vi "Sort 2D Array.vi"(8 "error in (no error)":errorcluster, 11 "Array in":string[][](array[string])) -> (0 "error out":errorcluster, 3 "Array out":string[][](array[string]))   [LabVIEW 2025, in "Project.lvclass"]
uses:
  Project.lvclass
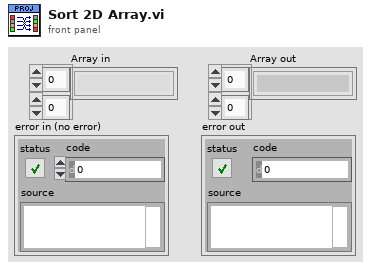
[diagram p1: front panel]
types:
  T1 = typedef "Project.lvclass/FPGA Settings.ctl" = cluster{"FPGA Target Name":string, "Modules":T2[]}
  T2 = typedef "Module.lvclass/Module Settings.ctl" = cluster{"Group Name":string, "Model Number":string, "Signals":T3[]}
  T3 = typedef "Signal.lvclass/Signal Settings.ctl" = cluster{"Signal Name":string, "IO Name":string, "Signal Type":string, "Signal Parameters":string, "IO Resource":string}
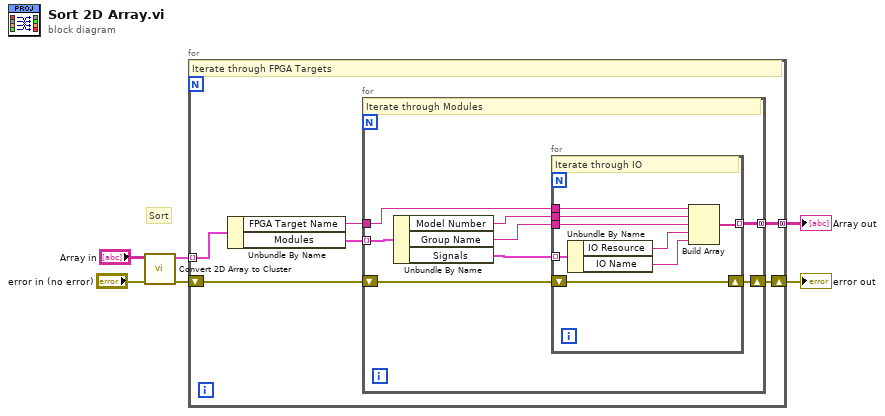
[diagram p0: block diagram]
diagram:
  # "Sort"
  n1 = call "Convert 2D Array to Cluster.vi"("error in (no error)"="error in (no error)", "Array in"="Array in") -> ("error out"=w3:errorcluster, "Array out"=w5:T1[])  [unwired: 8 in]
  n2 = for {
    tunnel: w5 -> [w10] mode=indexing
    shift-right: [w9] -> w1
    shift-left: w3 -> [w11]
    tunnel: [w7] -> w2 mode=concatenating
    # "Iterate through FPGA Targets"
    n3 = Unbundle By Name(w10) -> ("FPGA Target Name"=w8:string, "Modules"=w12:T2[])
    n4 = for {
      tunnel: w12 -> [w19] mode=indexing
      shift-right: [w18] -> w9
      shift-left: w11 -> [w13]
      tunnel: w8 -> [w17]
      tunnel: [w14] -> w7 mode=concatenating
      # "Iterate through Modules"
      n5 = Unbundle By Name(w19) -> ("Model Number"=w16:string, "Group Name"=w15:string, "Signals"=w20:T3[])
      n6 = for {
        tunnel: w20 -> [w21] mode=indexing
        shift-right: [w28] -> w18
        shift-left: w13 -> [w28]
        tunnel: w17 -> [w27]
        tunnel: w16 -> [w26]
        tunnel: w15 -> [w25]
        tunnel: [w22] -> w14 mode=indexing
        # "Iterate through IO"
        n7 = Unbundle By Name(w21) -> ("IO Resource"=w24:string, "IO Name"=w23:string)
        n8 = Build Array(w27, w26, w25, w24, w23) -> (w22:string[])
      }
    }
  }
  "Array out" <- w2
  "error out" <- w1
